vi "JSON Boolean To String.vi"(7 "enable LabVIEW extensions? (T)":bool=TRUE, 8 "error in (no error)":errorcluster, 11 "JSON Boolean in":refnum<class "JSON Helper.lvclass">) -> (0 "error out":errorcluster, 3 "String":string)   [LabVIEW 2016, in "JSON Helper.lvclass"]
uses:
  JSON Helper/JSON Helper.lvclass
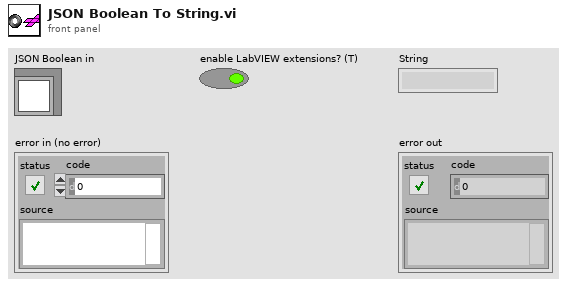
[diagram p1: front panel]
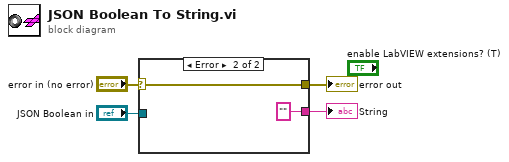
[diagram p0: block diagram]
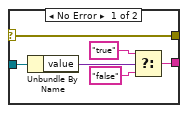
[diagram p2: hidden frame]
diagram:
  n1 = case shown="Error" "error in (no error)" {
    selector: "error in (no error)" -> [w5 w11]
    tunnel: "JSON Boolean in" -> [w10 _]
    tunnel: [w6 "" ("f")] -> w3
    tunnel: [w5 w11] -> w1
    frame No Error {
      n2 = Unbundle By Name(w10) -> ("value"=w9:variant)
      n3 = Select(t="true" ("String"), s=w9, f="false") -> (s? t:f=w6:string)
    }
    frame Error {
    }
  }
  "String" <- w3
  "error out" <- w1
